vi "VFH-file_handle-convert_r140.vi"(7 "Xi":dbl[](array[numeric]), 10 "file path (dialog if empty)":path=path "C:/projects/Universitet/Master/data/Initial Measurement Data/20240730/R140/Vann men kalib.xlsx") -> (2 "Handled data":T1)   [LabVIEW 2020, in "VFH-VNA_File_Handler.lvlib"]
uses:
  VFH-VNA_File_Handler.lvlib
  VFH-file_cluster-r140.ctl
panel:
  out "Waveform Graph":dbl[](graph)
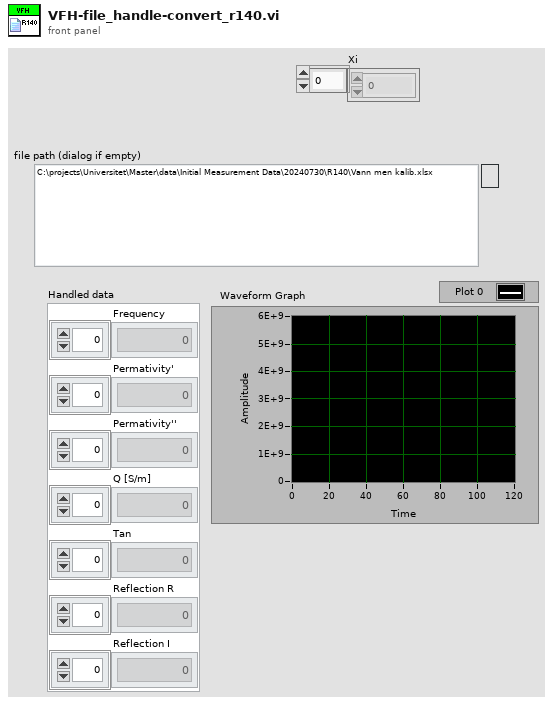
[diagram p1: front panel]
types:
  T1 = typedef "VFH-VNA_File_Handler.lvlib/VFH-file_cluster-r140.ctl" = cluster{"Frequency":dbl[], "Permativity'":dbl[], "Permativity''":dbl[], "Q [S/m]":dbl[], "Tan":dbl[], "Reflection R":dbl[], "Reflection I":dbl[]}
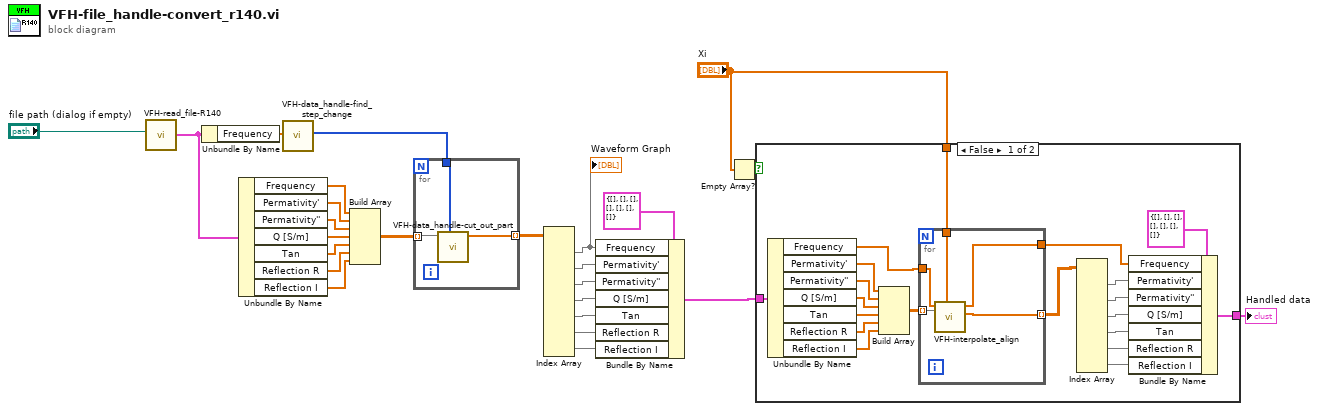
[diagram p0: block diagram]
diagram:
  n1 = call "VFH-read_file-R140.vi"("file path (dialog if empty)"="file path (dialog if empty)") -> ("Read data"=w25:T1)  [unwired: 8 in, 2 out]
  n2 = Unbundle By Name(w25) -> ("Frequency"=w6:dbl[])
  n3 = Unbundle By Name(w25) -> ("Frequency"=w23:dbl[], "Permativity'"=w22:dbl[], "Permativity''"=w21:dbl[], "Q [S/m]"=w20:dbl[], "Tan"=w19:dbl[], "Reflection R"=w18:dbl[], "Reflection I"=w17:dbl[])
  n4 = call "VFH-data_handle-find_step_change.vi"("data"=w6) -> ("step points"=w5:i32[])  [unwired: 10 in]
  n5 = Build Array(w23, w22, w21, w20, w19, w18, w17) -> (w16:dbl[][])
  n6 = for {
    tunnel: w16 -> [w28] mode=indexing
    tunnel: w5 -> [w27]
    tunnel: [w26] -> w15 mode=indexing
    n7 = call "VFH-data_handle-cut_out_part.vi"("Start and stop"=w27, "data"=w28) -> ("handled Data"=w26:dbl[])  [unwired: 8 in, 1 out]
  }
  n8 = Index Array(array=w15) -> (element #1=w8:dbl[], element #2=w14:dbl[], element #3=w13:dbl[], element #4=w12:dbl[], element #5=w11:dbl[], element #6=w10:dbl[], element #7=w9:dbl[])  [unwired: 14 in]
  "Waveform Graph" <- w8
  n9 = Bundle By Name(cluster=T1 {"Frequency"=[], "Permativity'"=[], "Permativity''"=[], "Q [S/m]"=[], "Tan"=[], "Reflection R"=[], "Reflection I"=[]} ("output cluster"), "Frequency"=w8, "Permativity'"=w14, "Permativity''"=w13, "Q [S/m]"=w12, "Tan"=w11, "Reflection R"=w10, "Reflection I"=w9) -> (w4:T1)
  n10 = Empty Array?(array="Xi") -> (empty?=w1:bool)
  n11 = case shown="False" w1 {
    tunnel: "Xi" -> [w40 _]
    tunnel: w4 -> [w39 w54]
    tunnel: [w29 w54] -> w3
    frame False {
      n12 = Unbundle By Name(w39) -> ("Frequency"=w41:dbl[], "Permativity'"=w48:dbl[], "Permativity''"=w47:dbl[], "Q [S/m]"=w46:dbl[], "Tan"=w45:dbl[], "Reflection R"=w44:dbl[], "Reflection I"=w43:dbl[])
      n13 = Build Array(w48, w47, w46, w45, w44, w43) -> (w42:dbl[][])
      n14 = for {
        tunnel: w42 -> [w53] mode=indexing
        tunnel: w41 -> [w52]
        tunnel: w40 -> [w51]
        tunnel: [w50] -> w32 mode=indexing
        tunnel: [w49] -> w30
        n15 = call "VFH-interpolate_align.vi"("Xi"=w51, "data"=w53, "Frequency"=w52) -> ("data out"=w50:dbl[], "Frequency out"=w49:dbl[])  [unwired: 7 in]
      }
      n16 = Index Array(array=w32) -> (element #1=w33:dbl[], element #2=w34:dbl[], element #3=w35:dbl[], element #4=w36:dbl[], element #5=w37:dbl[], element #6=w38:dbl[])  [unwired: 12 in]
      n17 = Bundle By Name(cluster=T1 {"Frequency"=[], "Permativity'"=[], "Permativity''"=[], "Q [S/m]"=[], "Tan"=[], "Reflection R"=[], "Reflection I"=[]} ("output cluster"), "Frequency"=w30, "Permativity'"=w33, "Permativity''"=w34, "Q [S/m]"=w35, "Tan"=w36, "Reflection R"=w37, "Reflection I"=w38) -> (w29:T1)
    }
    frame True {
    }
  }
  "Handled data" <- w3
